vi "DMA.Read Block.vi"(8 "error in (no error)":errorcluster, 10 "block index":i32, 11 "GE 5565 params":T1 {"DMA Blocks"."size" format="%08x"; "DMA Blocks"."pointer" format="%08x"}) -> (0 "error out":errorcluster, 1 "data":dbl[](array[numeric]), 2 "block index out":i32, 3 "GE 5565 params out":T1 {"DMA Blocks"."size" format="%08x"; "DMA Blocks"."pointer" format="%08x"})   [LabVIEW 2016, in "GE 5565PIORC.lvclass"]
uses:
  GE 5565PIORC.lvclass
  Controls/GE 5565 Params.ctl
  Controls/DMA Block.ctl
  Controls/DMA Config.ctl
  <vilib>/Instr/_visa.llb/VISA Register Access Address Space.ctl
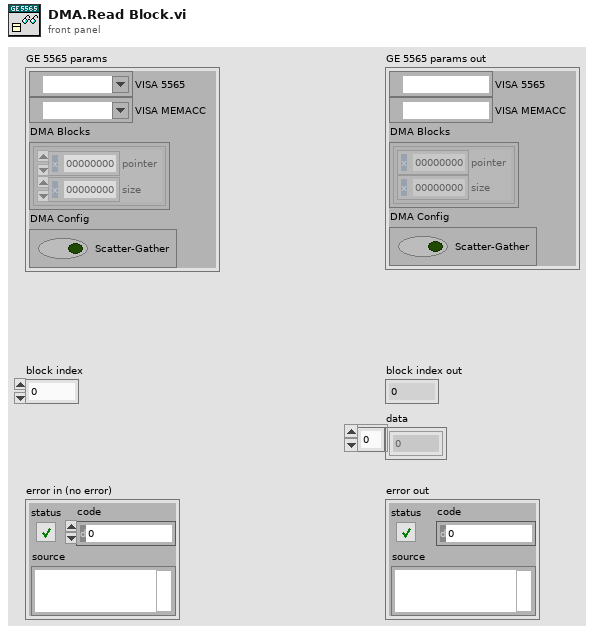
[diagram p1: front panel]
types:
  T1 = typedef "GE 5565PIORC.lvclass/GE 5565 Params.ctl" = cluster{"VISA 5565":refnum<visa-resource-name>, "VISA MEMACC":refnum<visa-resource-name>, "DMA Blocks":T2[], "DMA Config":T3}
  T2 = typedef "GE 5565PIORC.lvclass/DMA Block.ctl" = cluster{"pointer":u32, "size":u32}
  T3 = typedef "GE 5565PIORC.lvclass/DMA Config.ctl" = cluster{"Scatter-Gather":bool}
  T4 = typedef "VISA Register Access Address Space.ctl" = u16
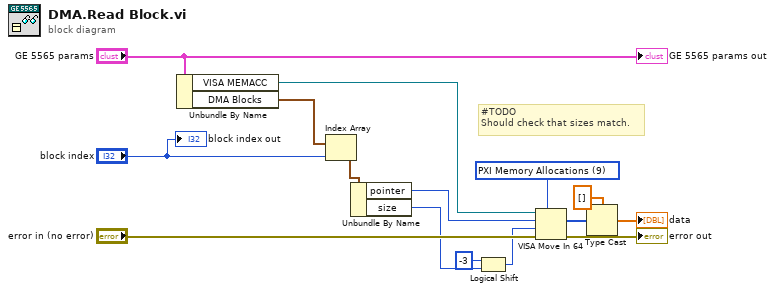
[diagram p0: block diagram]
diagram:
  w14 = T4 9 items=["VXI/VME A16"=1, "VXI/VME A24"=2, "VXI/VME A32"=3, "VXI/VME A64"=4, "PXI Memory Allocations"=9, "PXI Configuration"=10, "PXI BAR0"=11, "PXI BAR1"=12, "PXI BAR2"=13, "PXI BAR3"=14, "PXI BAR4"=15, "PXI BAR5"=16] ("Address Space")
  # "#TODO\nShould check that sizes match."
  n1 = Unbundle By Name("GE 5565 params") -> ("VISA MEMACC"=w9:refnum<visa-resource-name>, "DMA Blocks"=w8:T2[])
  n2 = Index Array(array=w8, index="block index") -> (element=w12:T2)
  n3 = Unbundle By Name(w12) -> ("pointer"=w13:u32, "size"=w3:u32)
  n4 = Logical Shift(y=i16 -3, x=w3) -> (x << y=w1:u32)
  n5 = VISA Move In 64(7:w14, 8:"error in (no error)", 9:w1, 10:w13, 11:w9) -> (0:→"error out":errorcluster, 2:w6:u64[])  [unwired: 1 out]
  n6 = Type Cast(type=dbl[] [] ("initialized array"), x=w6) -> (*(type *) &x=→"data":dbl[])
  "GE 5565 params out" <- "GE 5565 params"
  "block index out" <- "block index"
